vi "CheckIfReady.vi"(10 "Message Cluster in":T2, 11 "Enum":T1(ring)) -> (3 "Message Cluster out":T2)   [LabVIEW 2018]
doc: "Controlla che lo stato sia effettivamente ready"
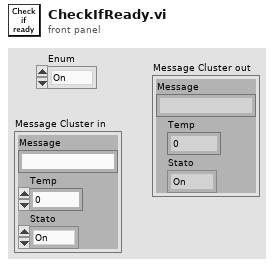
[diagram p1: front panel]
types:
  T1 = enum16{"On", "Off", "Preparation", "WaitTimer", "Ready"}
  T2 = cluster{"Message":string, "Temp":i32, "Stato":enum16{"On", "Off", "Preparation", "WaitTimer", "Ready"}}
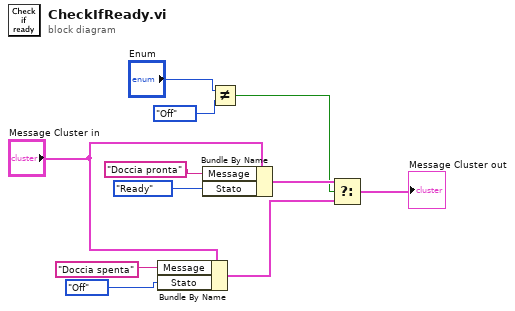
[diagram p0: block diagram]
diagram:
  n1 = Bundle By Name(cluster="Message Cluster in", "Message"="Doccia spenta", "Stato"=T1."Off") -> (w11:T2)
  n2 = Bundle By Name(cluster="Message Cluster in", "Message"="Doccia pronta", "Stato"=T1."Ready") -> (w6:T2)
  n3 = Not Equal?(x="Enum", y=T1."Off") -> (x != y?=w1:bool)
  n4 = Select(t=w6, s=w1, f=w11) -> (s? t:f=→"Message Cluster out":T2)
